vi "Transmit and Receive List Buffers.vi"() -> ()   [LabVIEW 2019]
doc: "The example program opens the specified Card and Core, and loads the provided\nXML configuration files. The XML configures a transmit channel, schedules a single \nmessage and configures a receive channel with self-test wraparound enabled. Both \nchannels are buffered through lists, which guarantee that all values for that label are \nseen before they get overwritten."
uses:
  <instrlib>/BTICardLib/Private/Initialize By Card Number and Core Number.vi
  <instrlib>/BTICardLib/Private/Configure Core From XML.vi
  <instrlib>/BTI429Lib/Private/Tx/Configure/Configure Tx Channel From XML.vi
  <instrlib>/BTI429Lib/Private/Rx/Configure/Configure Rx Channel From XML.vi
  <instrlib>/BTI429Lib/Private/Rx/Configure/Get Rx Label Handle Name.vi
  <instrlib>/BTI429Lib/Private/Core/Action-Status/Start All Channels.vi
  <instrlib>/BTI429Lib/Private/Core/Action-Status/Stop All Channels.vi
  <instrlib>/BTICardLib/BTICardLV.lvlib
  <instrlib>/BTI429Lib/BTI429LV.lvlib
panel:
  out "tx channel number":i32
  out "rx channel number":i32
  out "core number":i32
  in  "Rx Channel XML Configuration File":string="Rx Channel Config.xml"
  out "RCV Airspeed":u32 format="%08x"
  in  "stop":bool
  out "error out":errorcluster
  in  "Card Number":i32
  in  "Tx Channel XML Configuration File":string="Tx Channel Config.xml"
  in  "Core XML Configuration File":string="Core Config.xml"
  # "ARINC 429: Transmit and Receive List Buffers"
  # "©2016 Astronics Ballard Technology"
  # "The example program opens the specified Card and Core, and loads the provided\nXML configuration files. The XML configures a transmit channel, schedules a single \nmessage and configures a receive channel with self-test wraparound enabled. Both \nchannels are buffered through lists, which guarantee that all values for that label are \nseen before they get overwritten."
  # "Always Stop the card\nand Close the card when\ndone. Otherwise, the hardware\ncontinues to operate."
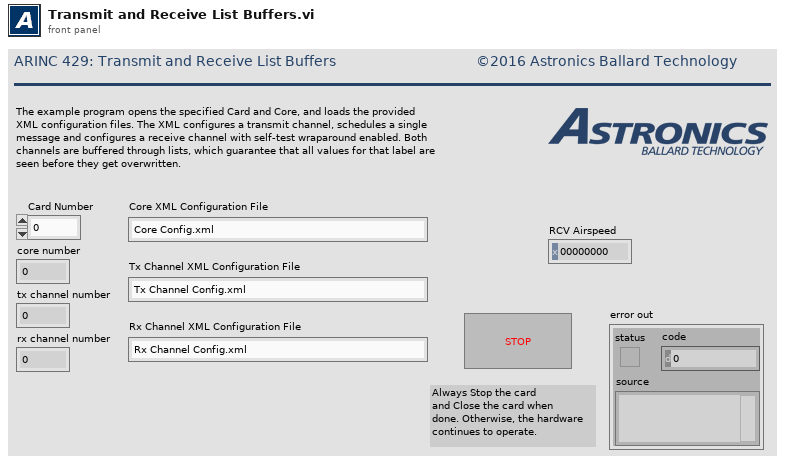
[diagram p1: front panel]
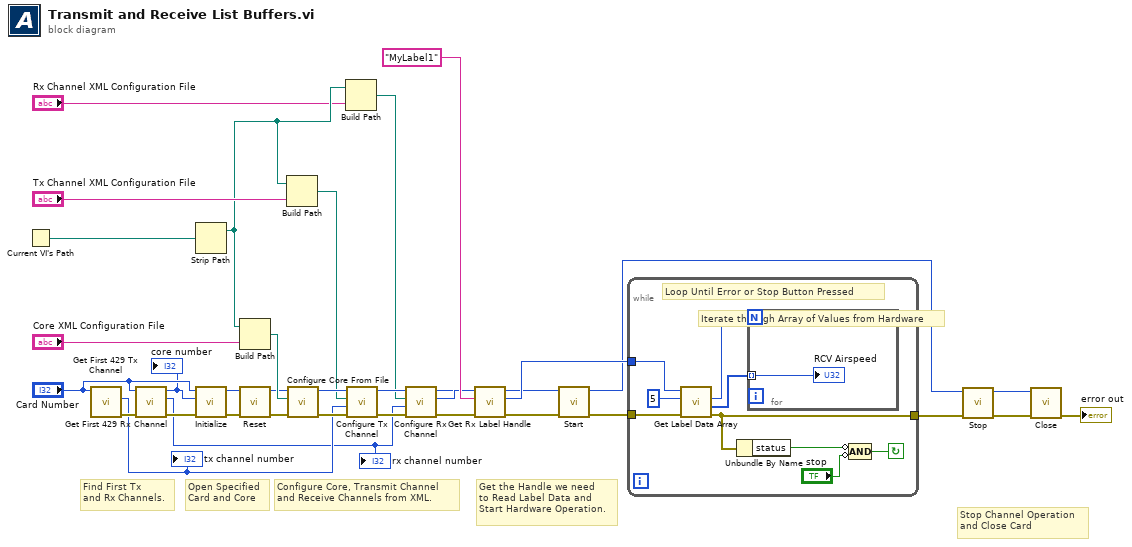
[diagram p0: block diagram]
diagram:
  # "Find First Tx \nand Rx Channels."
  # "Get the Handle we need\nto Read Label Data and \nStart Hardware Operation."
  # "Configure Core, Transmit Channel\nand Receive Channels from XML."
  # "Open Specified\nCard and Core"
  # "Stop Channel Operation\nand Close Card"
  n1 = Current VI's Path() -> (path=w24:path)
  n2 = call "Get First 429 Tx Channel.vi"("Card Number"="Card Number") -> ("error out"=w3:errorcluster, "Channel Number"=w2:i32)  [unwired: 8 in, 1 out]
  "tx channel number" <- w2
  n3 = call "Get First 429 Rx Channel.vi"("error in (no error)"=w3, "Card Number"="Card Number") -> ("error out"=w4:errorcluster, "Channel Number"=w1:i32, "Core Number"=w5:i32)  [unwired: 7 in]
  "core number" <- w5
  "rx channel number" <- w1
  n4 = Strip Path(path=w24) -> (stripped path=w16:path)  [unwired: 1 out]
  n5 = call-poly <instrlib>:"Initialize.vi"("error in (no error)"=w4, "core number"=w5, "card number"="Card Number") -> ("error out"=w7:errorcluster, "core handle out"=w10:u64)  [unwired: 7 in]
  n6 = Build Path(base path=w16, name or relative path="Core XML Configuration File") -> (appended path=w22:path)
  n7 = call <instrlib>:"Reset.vi"("error in (no error)"=w7, "core handle in"=w10) -> ("error out"=w8:errorcluster, "core handle out"=w9:u64)  [unwired: 8 in]
  n8 = Build Path(base path=w16, name or relative path="Tx Channel XML Configuration File") -> (appended path=w20:path)
  n9 = call-poly <instrlib>:"Configure Core From File.vi"("error in (no error)"=w8, "configuration file path"=w22, "core handle in"=w9) -> ("error out"=w33:errorcluster, "core handle out"=w34:u64)  [unwired: 7 in]
  n10 = Build Path(base path=w16, name or relative path="Rx Channel XML Configuration File") -> (appended path=w17:path)
  n11 = call-poly <instrlib>:"Configure Tx Channel.vi"("error in (no error)"=w33, "channel number in"=w2, "configuration file path"=w20, "core handle in"=w34) -> ("error out"=w13:errorcluster, "core handle out"=w19:u64)  [unwired: 5 in, 1 out]
  n12 = call-poly <instrlib>:"Configure Rx Channel.vi"("error in (no error)"=w13, "channel number in"=w1, "configuration file path"=w17, "core handle in"=w19) -> ("error out"=w12:errorcluster, "channel handle out"=w18:u64, "core handle out"=w14:u64)  [unwired: 5 in]
  n13 = call-poly <instrlib>:"Get Rx Label Handle.vi"("error in (no error)"=w12, "label name"="MyLabel1", "channel handle in"=w18) -> ("error out"=w31:errorcluster, "label handle out"=w28:u64)  [unwired: 6 in, 1 out]
  n14 = call-poly <instrlib>:"Start.vi"("error in (no error)"=w31, "core handle in"=w14) -> ("error out"=w30:errorcluster, "core handle out"=w25:u64)  [unwired: 8 in]
  n15 = while {
    tunnel: [w40] -> w32
    tunnel: w30 -> [w36]
    tunnel: w28 -> [w35]
    stop <- w43 continue-if-true
    # "Loop Until Error or Stop Button Pressed"
    n16 = call <instrlib>:"Get Label Data Array.vi"("error in (no error)"=w36, "data items to read"=u32 5, "label handle in"=w35) -> ("error out"=w40:errorcluster, "data values"=w38:u32[], "data items read"=w39:u32)  [unwired: 5 in, 1 out]
    n17 = Unbundle By Name(w40) -> ("status"=w41:bool)
    n18 = for {
      N: w39 -> [_]
      tunnel: w38 -> [w44] mode=indexing
      # "Iterate through Array of Values from Hardware"
      "RCV Airspeed" <- w44
    }
    n19 = Compound Arithmetic op=AND(invert w41, invert "stop") -> (w43:bool)
  }
  n20 = call-poly <instrlib>:"Stop.vi"("error in (no error)"=w32, "core handle in"=w25) -> ("error out"=w27:errorcluster, "core handle out"=w11:u64)  [unwired: 8 in]
  n21 = call <instrlib>:"Close.vi"("error in (no error)"=w27, "core handle in"=w11) -> ("error out"=→"error out":errorcluster)  [unwired: 8 in, 1 out]
